vi "Event Read.vi"(11 "Event Registration Refnum in":refnum<event-registration>) -> (2 "Quit":bool, 3 "value":bool)   [LabVIEW 2021]
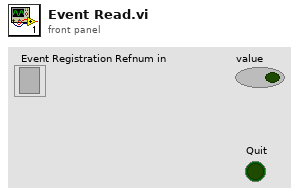
[diagram p1: front panel]
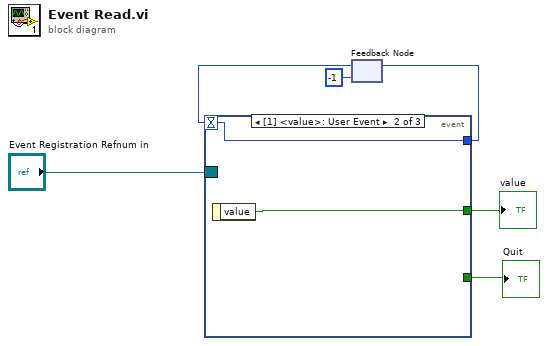
[diagram p0: block diagram]
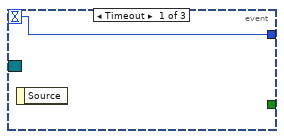
[diagram p2: hidden frame]
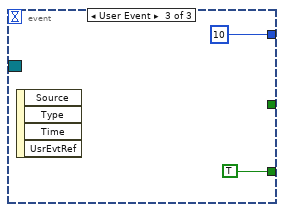
[diagram p3: hidden frame]
diagram:
  n1 = feedback #1(-1) -> (w3:i32)
  n2 = event shown="[1] <value>: User Event" {
    selector: "Event Registration Refnum in" -> [_ _ _]
    dyn-events: _ -> [_ _ _]
    timeout: w3 -> [w7 w9 _]
    tunnel: [w7 w9 10] -> w4
    tunnel: [_ w8 _] -> w6
    tunnel: [_ _ TRUE] -> w1
    event Timeout {
      n3 = event-data() -> ()  [unwired: 1 in, 1 out]
    }
    event User Event {
      n4 = event-data() -> ("value"=w8:bool)  [unwired: 1 in]
    }
    event User Event {
      n5 = event-data() -> ()  [unwired: 1 in, 4 out]
    }
  }
  "value" <- w6
  "Quit" <- w1
  n6 = feedback-in #1(w4) -> ()
